vi "Begin.vi"(8 "error in":errorcluster) -> (0 "error out":errorcluster)   [LabVIEW 2020]
doc: "Called before other user functions, this VI can be used to open I/O refnums, load in file data, and do general program initialization. Notice that the <B>error out</B> terminal is simply used for data flow. Wiring it to other structures or subVIs ensures that this VI runs first."
uses:
  <vilib>/Rock Robotics/WPI/DriverStation/WPI_DriverStationRobotMode2.ctl
  <vilib>/Rock Robotics/WPI/Joystick/WPI_JoystickDeviceEnum.ctl
  <vilib>/Rock Robotics/WPI/SafetyOutput/WPI_SafetyOutputConfigMenu.ctl
  <vilib>/Rock Robotics/WPI/ThirdParty/REV Robotics/SPARK MAX/Typedef/Spark MAX Idle Mode.ctl
  <vilib>/Rock Robotics/SystemInterfaces/DIO/FPGA_DIOChannel.ctl
  <vilib>/Rock Robotics/WPI/Solenoid/WPI_SolenoidChannel.ctl
  <vilib>/Rock Robotics/WPI/Solenoid/WPI_SolenoidValue.ctl
  <vilib>/Rock Robotics/SystemInterfaces/DIO/FPGA_DIOPWMChannel.ctl
  Robot Global Data.vi
  <vilib>/Rock Robotics/Network Tables/NT Write String Array.vi
  <vilib>/Rock Robotics/WPI/Solenoid/WPI_SolenoidOpenDouble.vi
  <vilib>/Rock Robotics/WPI/Utilities/WPI_GetSetVariantRefNum.vi
  <vilib>/Rock Robotics/WPI/Solenoid/WPI_SolenoidSetEnum.vi
  <vilib>/Rock Robotics/WPI/MotorControl/WPI_MotorControlOpen SPARK.vi
  <vilib>/Rock Robotics/WPI/MotorControl/WPI_MotorControlOpen VictorSPX.vi
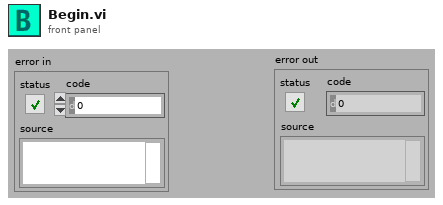
[diagram p1: front panel]
types:
  T1 = typedef "FPGA_DIOPWMChannel.ctl" = enum8{"PWM 0", "PWM 1", "PWM 2", "PWM 3", "PWM 4", "PWM 5", "PWM 6", "PWM 7", "PWM 8", "PWM 9", "PWM MXP 0", "PWM MXP 1", "PWM MXP 2", "PWM MXP 3", "PWM MXP 4", "PWM MXP 5", "PWM MXP 6", "PWM MXP 7", "PWM MXP 8", "PWM MXP 9", "Invalid"}
  T2 = typedef "WPI_SafetyOutputConfigMenu.ctl" = enum16{"Enable", "Disable"}
  T3 = typedef "WPI_SolenoidValue.ctl" = enum16{"Off", "On", "Forward", "Reverse"}
  T4 = typedef "WPI_SolenoidChannel.ctl" = enum8{"Solenoid 0", "Solenoid 1", "Solenoid 2", "Solenoid 3", "Solenoid 4", "Solenoid 5", "Solenoid 6", "Solenoid 7", "Solenoid 8", "Solenoid 9", "Solenoid 10", "Solenoid 11", "Solenoid 12", "Solenoid 13", "Solenoid 14", "Solenoid 15", "Invalid"}
  T5 = typedef "Spark MAX Idle Mode.ctl" = enum16{"Coast", "Brake"}
  T6 = typedef "FPGA_DIOChannel.ctl" = enum8{"DIO 0", "DIO 1", "DIO 2", "DIO 3", "DIO 4", "DIO 5", "DIO 6", "DIO 7", "DIO 8", "DIO 9", "DIO MXP 0", "DIO MXP 1", "DIO MXP 2", "DIO MXP 3", "DIO MXP 4", "DIO MXP 5", "DIO MXP 6", "DIO MXP 7", "DIO MXP 8", "DIO MXP 9", "DIO MXP 10", "DIO MXP 11", "DIO MXP 12", "DIO MXP 13", "DIO MXP 14", "DIO MXP 15", "SPI Port CS1", "SPI Port CS2", "SPI Port CS3", "SPI Port MISO", "SPI Port MOSI", "Invalid"}
  T7 = typedef "WPI_JoystickDeviceEnum.ctl" = enum16{"USB 0", "USB 1", "USB 2", "USB 3", "USB 4", "USB 5"}
  T8 = typedef "WPI_DriverStationRobotMode2.ctl" = enum16{"Autonomous Disabled", "Autonomous Enabled", "Teleop Disabled", "Teleop Enabled", "Disconnected", "Finish", "Test Disabled", "Test Enabled", "Emergency Stopped"}
  T9 = typedef "WPI_MotorControlDeviceRef.ctl" = cluster{"DeviceStatus":errorcluster, "Type":T10, "PWM":cluster{"PWM Channel":T1, "DeadBand":T11}, "CAN":cluster{"Device Number":u8, "SetOutput VI Ref":variant, "GetOutput VI Ref":variant, "Enable VI Ref":variant, "Disable VI Ref":variant, "Data":variant}, "Invert":bool, "DIO PWM":cluster{"PWM \"Enable\" Channel":T1, "DIOChannel":T6, "PWM Rate":dbl}}
  T10 = typedef "WPI_MotorControlType.ctl" = enum16{"PWM", "CAN", "DIO PWM"}
  T11 = typedef "WPI_PWMDeadband.ctl" = cluster{"Name":string, "maxPositivePwm":i32, "minPositivePwm":i32, "centerPwm":i32, "maxNegativePwm":i32, "minNegativePwm":i32, "angularRange":u16}
  T12 = typedef "WPI_SolenoidDevRef.ctl" = cluster{"DevStatus":errorcluster, "Pneumatics Control Module":u8, "Forward Solenoid Channel":T4, "Reverse Solenoid Channel":T4}
  T13 = typedef "WPI_JoystickDevRef.ctl" = cluster{"Device":T7}
  T14 = typedef "ADIS16470 Device Reference.ctl" = cluster{"DevStatus":errorcluster, "Hardware Config":T15, "Calibration Complete":refnum<notifier>, "Status Reference":refnum<data-value>, "Data Reference":refnum<data-value>, "Sychronous Process VI":T18, "Cmd FIFO":refnum<k33>, "Source":T19, "Data FIFO":refnum<k33>, "Calibration Time (ms)":u32, "Data Reference":refnum<data-value>}
  T15 = typedef "ADIS16470 Hardware Configuration.ctl" = cluster{"SPI Clock Rate (Hz)":dbl, "IMU SPI Mode (3)":T16, "IMU Reset Pin":T6, "IMU SPI Bus":T17, "IMU Data Ready Pin":T6, "Stall Config":cluster{"Pow2BytesPerRead":u8, "StallTicks":u16, "CsToSclkTicks":u8}}
  T16 = typedef "WPI_SPIMode.ctl" = enum16{"Mode 0 (Clk Idle Low,Sample on Leading)", "Mode 1 (Clk Idle Low,Sample on Trailing)", "Mode 2 (Clk Idle High,Sample on Leading)", "Mode 3 (Clk Idle High,Sample on Trailing)"}
  T17 = typedef "spi_bus.ctl" = enum16{"SPI On-Board, CS0", "SPI On-Board, CS1", "SPI On-Board, CS2", "SPI On-Board, CS3", "SPI MXP", "Invalid"}
  T18 = typedef "ADIS16470 Process.ctl" = refnum<vi>
  T19 = typedef "FPGA_CounterEncoderSourceConvertionLVSourceType.ctl" = cluster{"DevStatus":errorcluster, "AnalogTriggerMode?":bool, "DigitalMode":cluster{"DIO Channel":T20}, "AnalogTriggerMode":cluster{"AnalogTriggerIndex":T21, "OutputType":T22}}
  T20 = typedef "FPGA_DIODigitalSourceChannel.ctl" = enum8{"DIO 0", "DIO 1", "DIO 2", "DIO 3", "DIO 4", "DIO 5", "DIO 6", "DIO 7", "DIO 8", "DIO 9", "DIO MXP 0", "DIO MXP 1", "DIO MXP 2", "DIO MXP 3", "DIO MXP 4", "DIO MXP 5", "DIO MXP 6", "DIO MXP 7", "DIO MXP 8", "DIO MXP 9", "DIO MXP 10", "DIO MXP 11", "DIO MXP 12", "DIO MXP 13", "DIO MXP 14", "DIO MXP 15", "SPI Port CS1", "SPI Port CS2", "SPI Port CS3", "SPI Port MISO", "SPI Port MOSI", "Disabled"}
  T21 = typedef "FPGA_AnalogTriggerIndex.ctl" = enum8{"Trig 0", "Trig 1", "Trig 2", "Trig 3", "Trig 4", "Trig 5", "Trig 6", "Trig 7", "Invalid"}
  T22 = typedef "FPGA_AnalogTriggerOutType.ctl" = enum16{"InWindow", "TriggerState", "Rising", "Falling"}
  T23 = typedef "WPI_DigitalInputDevRef.ctl" = cluster{"DevStatus":errorcluster, "DIO Channel":T6}
  T24 = typedef "WPI_CompressorDevRef.ctl" = cluster{"DevStatus":errorcluster, "Pneumatics Control Module":u8}
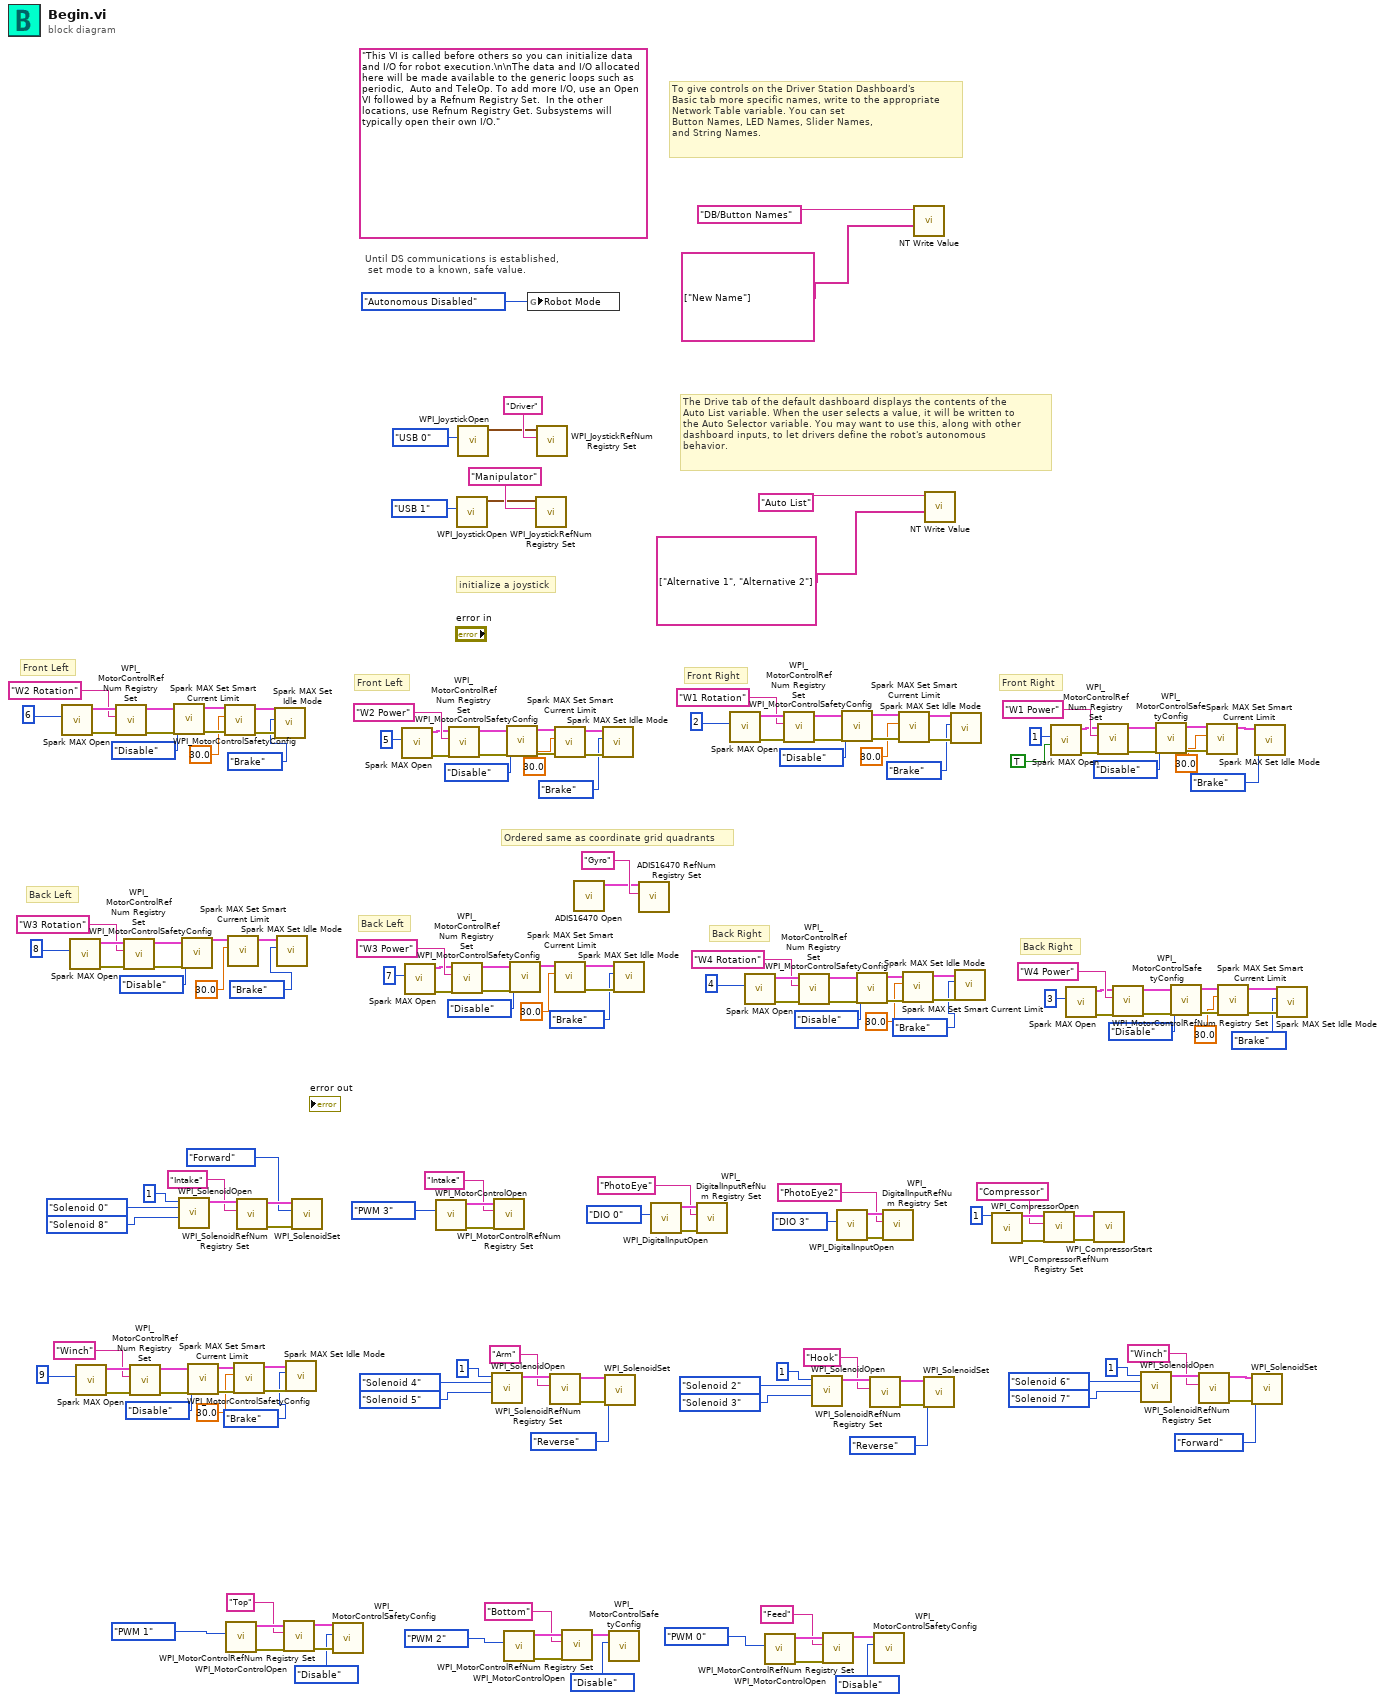
[diagram p0: block diagram]
diagram:
  (unwired) "This VI is called before others so you can initialize data and I/O for robot execution.\n\nThe data and I/O allocated here will be made available to the generic loops such as periodic,  Auto and TeleOp. To add more I/O, use an Open VI followed by a Refnum Registry Set.  In the other locations, use Refnum Registry Get. Subsystems will typically open their own I/O."
  # "Ordered same as coordinate grid quadrants"
  # "Back Right"
  # "Back Right"
  # "Back Left"
  # "Back Left"
  # "Front Left"
  # "Front Left"
  # "Front Right"
  # "Front Right"
  # "The Drive tab of the default dashboard displays the contents of the\nAuto List variable. When the user selects a value, it will be written to\nthe Auto Selector variable. You may want to use this, along with other\ndashboard inputs, to let drivers define the robot's autonomous\nbehavior."
  # "To give controls on the Driver Station Dashboard's\nBasic tab more specific names, write to the appropriate\nNetwork Table variable. You can set\nButton Names, LED Names, Slider Names,\nand String Names."
  # "initialize a joystick"
  # "Until DS communications is established,\n set mode to a known, safe value."
  n1 = call <vilib>:"Spark MAX Open.vi"("Device Number"=u8 6) -> ("error out"=w172:errorcluster, "MotorControlDeviceRef"=w171:T9)  [unwired: 9 in]
  n2 = call <vilib>:"Spark MAX Open.vi"("Device Number"=u8 8) -> ("error out"=w160:errorcluster, "MotorControlDeviceRef"=w159:T9)  [unwired: 9 in]
  n3 = call <vilib>:"Spark MAX Open.vi"("Device Number"=u8 9) -> ("error out"=w68:errorcluster, "MotorControlDeviceRef"=w67:T9)  [unwired: 9 in]
  n4 = call <vilib>:"WPI_MotorControlRefNum Registry Set.vi"("error in (no error)"=w172, "refnum name"="W2 Rotation", "MotorControlDevRef"=w171) -> ("error out"=w170:errorcluster, "MotorControlDevRef"=w108:T9)  [unwired: 7 in]
  n5 = call <vilib>:"WPI_MotorControlRefNum Registry Set.vi"("error in (no error)"=w160, "refnum name"="W3 Rotation", "MotorControlDevRef"=w159) -> ("error out"=w158:errorcluster, "MotorControlDevRef"=w157:T9)  [unwired: 7 in]
  n6 = call <vilib>:"WPI_MotorControlRefNum Registry Set.vi"("error in (no error)"=w68, "refnum name"="Winch", "MotorControlDevRef"=w67) -> ("error out"=w66:errorcluster, "MotorControlDevRef"=w65:T9)  [unwired: 7 in]
  n7 = call <vilib>:"WPI_MotorControlSafetyConfig.vi"("error in (no error)"=w170, "mode"=WPI_SafetyOutputConfigMenu."Disable", "MotorControlDevRef"=w108) -> ("error out"=w111:errorcluster, "MotorControlDevRef"=w110:T9)  [unwired: 7 in]
  n8 = call-poly <vilib>:"WPI_SolenoidOpen.vi"("Reverse Solenoid Channel"=WPI_SolenoidChannel."Solenoid 8", "Forward Solenoid Channel"=WPI_SolenoidChannel."Solenoid 0", "Pneumatics Device (def)"=u8 1) -> ("SolenoidDevRef"=w81:T12)  [unwired: 7 in, 1 out]
  n9 = call <vilib>:"WPI_MotorControlSafetyConfig.vi"("error in (no error)"=w158, "mode"=WPI_SafetyOutputConfigMenu."Disable", "MotorControlDevRef"=w157) -> ("MotorControlDevRef"=w130:T9)  [unwired: 7 in, 1 out]
  n10 = call <vilib>:"WPI_MotorControlSafetyConfig.vi"("error in (no error)"=w66, "mode"=WPI_SafetyOutputConfigMenu."Disable", "MotorControlDevRef"=w65) -> ("error out"=w61:errorcluster, "MotorControlDevRef"=w60:T9)  [unwired: 7 in]
  n11 = call <vilib>:"Spark MAX Set Smart Current Limit.vi"("error in (no error)"=w111, "Primay Current Limit (80A)"=30.0, "MotorControlDeviceRef in"=w110) -> ("error out"=w96:errorcluster, "MotorControlDeviceRef out"=w95:T9)  [unwired: 7 in]
  n12 = call-poly <vilib>:"WPI_MotorControlOpen.vi"("PWM Channel"=FPGA_DIOPWMChannel."PWM 1") -> ("error out"=w20:errorcluster, "MotorControlDeviceRef"=w19:T9)  [unwired: 9 in]
  n13 = call <vilib>:"Spark MAX Set Smart Current Limit.vi"("Primay Current Limit (80A)"=30.0, "MotorControlDeviceRef in"=w130) -> ("MotorControlDeviceRef out"=w97:T9)  [unwired: 8 in, 1 out]
  n14 = call <vilib>:"Spark MAX Set Smart Current Limit.vi"("error in (no error)"=w61, "Primay Current Limit (80A)"=30.0, "MotorControlDeviceRef in"=w60) -> ("error out"=w58:errorcluster, "MotorControlDeviceRef out"=w57:T9)  [unwired: 7 in]
  n15 = call <vilib>:"WPI_SolenoidRefNum Registry Set.vi"("refnum name"="Intake", "SolenoidDevRef"=w81) -> ("error out"=w32:errorcluster, "SolenoidDevRef"=w31:T12)  [unwired: 8 in]
  n16 = call <vilib>:"Spark MAX Set Idle Mode.vi"("error in (no error)"=w96, "Idle Mode"=Spark_MAX_Idle_Mode."Brake", "MotorControlDeviceRef in"=w95) -> ()  [unwired: 7 in, 2 out]
  n17 = call <vilib>:"Spark MAX Set Idle Mode.vi"("Idle Mode"=Spark_MAX_Idle_Mode."Brake", "MotorControlDeviceRef in"=w97) -> ()  [unwired: 8 in, 2 out]
  n18 = call <vilib>:"WPI_MotorControlRefNum Registry Set.vi"("error in (no error)"=w20, "refnum name"="Top", "MotorControlDevRef"=w19) -> ("error out"=w4:errorcluster, "MotorControlDevRef"=w3:T9)  [unwired: 7 in]
  n19 = call <vilib>:"Spark MAX Set Idle Mode.vi"("error in (no error)"=w58, "Idle Mode"=Spark_MAX_Idle_Mode."Brake", "MotorControlDeviceRef in"=w57) -> ()  [unwired: 7 in, 2 out]
  n20 = call-poly <vilib>:"WPI_SolenoidSet.vi"("error in (no error)"=w32, "Value"=WPI_SolenoidValue."Forward", "SolenoidDevRef"=w31) -> ()  [unwired: 7 in, 2 out]
  n21 = call <vilib>:"WPI_MotorControlSafetyConfig.vi"("error in (no error)"=w4, "mode"=WPI_SafetyOutputConfigMenu."Disable", "MotorControlDevRef"=w3) -> ()  [unwired: 7 in, 2 out]
  n22 = call <vilib>:"Spark MAX Open.vi"("Device Number"=u8 5) -> ("error out"=w162:errorcluster, "MotorControlDeviceRef"=w163:T9)  [unwired: 9 in]
  n23 = call <vilib>:"Spark MAX Open.vi"("Device Number"=u8 7) -> ("error out"=w149:errorcluster, "MotorControlDeviceRef"=w150:T9)  [unwired: 9 in]
  n24 = call-poly <vilib>:"WPI_MotorControlOpen.vi"("PWM Channel"=FPGA_DIOPWMChannel."PWM 3") -> ("error out"=w79:errorcluster, "MotorControlDeviceRef"=w78:T9)  [unwired: 9 in]
  n25 = call <vilib>:"WPI_MotorControlRefNum Registry Set.vi"("error in (no error)"=w162, "refnum name"="W2 Power", "MotorControlDevRef"=w163) -> ("error out"=w167:errorcluster, "MotorControlDevRef"=w166:T9)  [unwired: 7 in]
  n26 = call <vilib>:"WPI_MotorControlRefNum Registry Set.vi"("error in (no error)"=w149, "refnum name"="W3 Power", "MotorControlDevRef"=w150) -> ("error out"=w154:errorcluster, "MotorControlDevRef"=w153:T9)  [unwired: 7 in]
  n27 = call <vilib>:"WPI_JoystickOpen.vi"("JoystickDevice"=WPI_JoystickDeviceEnum."USB 1") -> ("JoystickDevRef"=w187:T13)  [unwired: 10 in]
  n28 = call <vilib>:"WPI_JoystickOpen.vi"("JoystickDevice"=WPI_JoystickDeviceEnum."USB 0") -> ("JoystickDevRef"=w194:T13)  [unwired: 10 in]
  n29 = call-poly <vilib>:"WPI_SolenoidOpen.vi"("Reverse Solenoid Channel"=WPI_SolenoidChannel."Solenoid 5", "Forward Solenoid Channel"=WPI_SolenoidChannel."Solenoid 4", "Pneumatics Device (def)"=u8 1) -> ("SolenoidDevRef"=w52:T12)  [unwired: 7 in, 1 out]
  n30 = call <vilib>:"WPI_MotorControlRefNum Registry Set.vi"("error in (no error)"=w79, "refnum name"="Intake", "MotorControlDevRef"=w78) -> ()  [unwired: 7 in, 2 out]
  n31 = call-poly <vilib>:"WPI_MotorControlOpen.vi"("PWM Channel"=FPGA_DIOPWMChannel."PWM 2") -> ("error out"=w16:errorcluster, "MotorControlDeviceRef"=w15:T9)  [unwired: 9 in]
  n32 = call <vilib>:"WPI_MotorControlSafetyConfig.vi"("error in (no error)"=w167, "mode"=WPI_SafetyOutputConfigMenu."Disable", "MotorControlDevRef"=w166) -> ("error out"=w114:errorcluster, "MotorControlDevRef"=w113:T9)  [unwired: 7 in]
  n33 = call <vilib>:"WPI_MotorControlSafetyConfig.vi"("error in (no error)"=w154, "mode"=WPI_SafetyOutputConfigMenu."Disable", "MotorControlDevRef"=w153) -> ("MotorControlDevRef"=w128:T9)  [unwired: 7 in, 1 out]
  n34 = global write "Robot Global Data.vi" "Robot Mode"(WPI_DriverStationRobotMode2."Autonomous Disabled" ("Robot Mode")) -> ()
  n35 = call <vilib>:"WPI_JoystickRefNum Registry Set.vi"("refnum name"="Manipulator", "JoystickDevRef"=w187) -> ()  [unwired: 8 in, 2 out]
  n36 = call <vilib>:"WPI_JoystickRefNum Registry Set.vi"("refnum name"="Driver", "JoystickDevRef"=w194) -> ()  [unwired: 8 in, 2 out]
  n37 = call <vilib>:"WPI_SolenoidRefNum Registry Set.vi"("refnum name"="Arm", "SolenoidDevRef"=w52) -> ("error out"=w29:errorcluster, "SolenoidDevRef"=w28:T12)  [unwired: 8 in]
  n38 = call <vilib>:"Spark MAX Set Smart Current Limit.vi"("error in (no error)"=w114, "Primay Current Limit (80A)"=30.0, "MotorControlDeviceRef in"=w113) -> ("error out"=w100:errorcluster, "MotorControlDeviceRef out"=w99:T9)  [unwired: 7 in]
  n39 = call <vilib>:"Spark MAX Set Smart Current Limit.vi"("Primay Current Limit (80A)"=30.0, "MotorControlDeviceRef in"=w128) -> ("error out"=w102:errorcluster, "MotorControlDeviceRef out"=w101:T9)  [unwired: 8 in]
  n40 = call <vilib>:"WPI_MotorControlRefNum Registry Set.vi"("error in (no error)"=w16, "refnum name"="Bottom", "MotorControlDevRef"=w15) -> ("MotorControlDevRef"=w5:T9)  [unwired: 7 in, 1 out]
  n41 = call <vilib>:"ADIS16470 Open.vi"() -> ("ADIS16470DevRef"=w83:T14)  [unwired: 10 in, 1 out]
  n42 = call <vilib>:"Spark MAX Set Idle Mode.vi"("error in (no error)"=w100, "Idle Mode"=Spark_MAX_Idle_Mode."Brake", "MotorControlDeviceRef in"=w99) -> ()  [unwired: 7 in, 2 out]
  n43 = call-poly <vilib>:"WPI_SolenoidSet.vi"("error in (no error)"=w29, "Value"=WPI_SolenoidValue."Reverse", "SolenoidDevRef"=w28) -> ()  [unwired: 7 in, 2 out]
  n44 = call <vilib>:"WPI_MotorControlSafetyConfig.vi"("mode"=WPI_SafetyOutputConfigMenu."Disable", "MotorControlDevRef"=w5) -> ()  [unwired: 8 in, 2 out]
  n45 = call <vilib>:"Spark MAX Set Idle Mode.vi"("error in (no error)"=w102, "Idle Mode"=Spark_MAX_Idle_Mode."Brake", "MotorControlDeviceRef in"=w101) -> ()  [unwired: 7 in, 2 out]
  n46 = call <vilib>:"ADIS16470 RefNum Registry Set.vi"("refnum name"="Gyro", "ADIS16470DevRef in"=w83) -> ()  [unwired: 8 in, 2 out]
  n47 = call <vilib>:"WPI_DigitalInputOpen.vi"("DIO Channel"=FPGA_DIOChannel."DIO 0") -> ("error out"=w76:errorcluster, "DigitalInputDevRef"=w75:T23)  [unwired: 9 in]
  n48 = call <vilib>:"WPI_DigitalInputRefNum Registry Set.vi"("error in (no error)"=w76, "refnum name"="PhotoEye", "DigitalInputDevRef"=w75) -> ()  [unwired: 7 in, 2 out]
  n49 = call <vilib>:"Spark MAX Open.vi"("Device Number"=u8 2) -> ("error out"=w185:errorcluster, "MotorControlDeviceRef"=w184:T9)  [unwired: 9 in]
  n50 = call <vilib>:"Spark MAX Open.vi"("Device Number"=u8 4) -> ("error out"=w147:errorcluster, "MotorControlDeviceRef"=w146:T9)  [unwired: 9 in]
  n51 = call-poly <vilib>:"WPI_MotorControlOpen.vi"("PWM Channel"=FPGA_DIOPWMChannel."PWM 0") -> ("error out"=w12:errorcluster, "MotorControlDeviceRef"=w11:T9)  [unwired: 9 in]
  n52 = call <vilib>:"WPI_MotorControlRefNum Registry Set.vi"("error in (no error)"=w185, "refnum name"="W1 Rotation", "MotorControlDevRef"=w184) -> ("error out"=w183:errorcluster, "MotorControlDevRef"=w182:T9)  [unwired: 7 in]
  n53 = call <vilib>:"WPI_MotorControlRefNum Registry Set.vi"("error in (no error)"=w147, "refnum name"="W4 Rotation", "MotorControlDevRef"=w146) -> ("error out"=w145:errorcluster, "MotorControlDevRef"=w144:T9)  [unwired: 7 in]
  n54 = call-poly <vilib>:"WPI_SolenoidOpen.vi"("Reverse Solenoid Channel"=WPI_SolenoidChannel."Solenoid 3", "Forward Solenoid Channel"=WPI_SolenoidChannel."Solenoid 2", "Pneumatics Device (def)"=u8 1) -> ("SolenoidDevRef"=w47:T12)  [unwired: 7 in, 1 out]
  n55 = call <vilib>:"WPI_MotorControlRefNum Registry Set.vi"("error in (no error)"=w12, "refnum name"="Feed", "MotorControlDevRef"=w11) -> ("MotorControlDevRef"=w7:T9)  [unwired: 7 in, 1 out]
  n56 = call <vilib>:"WPI_DigitalInputOpen.vi"("DIO Channel"=FPGA_DIOChannel."DIO 3") -> ("error out"=w72:errorcluster, "DigitalInputDevRef"=w71:T23)  [unwired: 9 in]
  n57 = call <vilib>:"WPI_MotorControlSafetyConfig.vi"("error in (no error)"=w183, "mode"=WPI_SafetyOutputConfigMenu."Disable", "MotorControlDevRef"=w182) -> ("error out"=w117:errorcluster, "MotorControlDevRef"=w116:T9)  [unwired: 7 in]
  n58 = call <vilib>:"WPI_MotorControlSafetyConfig.vi"("error in (no error)"=w145, "mode"=WPI_SafetyOutputConfigMenu."Disable", "MotorControlDevRef"=w144) -> ("error out"=w126:errorcluster, "MotorControlDevRef"=w125:T9)  [unwired: 7 in]
  n59 = call <vilib>:"WPI_SolenoidRefNum Registry Set.vi"("refnum name"="Hook", "SolenoidDevRef"=w47) -> ("error out"=w24:errorcluster, "SolenoidDevRef"=w25:T12)  [unwired: 8 in]
  n60 = call <vilib>:"WPI_MotorControlSafetyConfig.vi"("mode"=WPI_SafetyOutputConfigMenu."Disable", "MotorControlDevRef"=w7) -> ()  [unwired: 8 in, 2 out]
  n61 = call <vilib>:"WPI_DigitalInputRefNum Registry Set.vi"("error in (no error)"=w72, "refnum name"="PhotoEye2", "DigitalInputDevRef"=w71) -> ()  [unwired: 7 in, 2 out]
  n62 = call <vilib>:"Spark MAX Set Smart Current Limit.vi"("error in (no error)"=w117, "Primay Current Limit (80A)"=30.0, "MotorControlDeviceRef in"=w116) -> ("error out"=w92:errorcluster, "MotorControlDeviceRef out"=w91:T9)  [unwired: 7 in]
  n63 = call <vilib>:"Spark MAX Set Smart Current Limit.vi"("error in (no error)"=w126, "Primay Current Limit (80A)"=30.0, "MotorControlDeviceRef in"=w125) -> ("error out"=w90:errorcluster, "MotorControlDeviceRef out"=w89:T9)  [unwired: 7 in]
  n64 = call-poly <vilib>:"NT Write Value.vi"("String Array"=string[] ["New Name"], "Name"="DB/Button Names") -> ()  [unwired: 9 in, 1 out]
  n65 = call-poly <vilib>:"WPI_SolenoidSet.vi"("error in (no error)"=w24, "Value"=WPI_SolenoidValue."Reverse", "SolenoidDevRef"=w25) -> ()  [unwired: 7 in, 2 out]
  n66 = call-poly <vilib>:"NT Write Value.vi"("String Array"=string[] ["Alternative 1", "Alternative 2"], "Name"="Auto List") -> ()  [unwired: 9 in, 1 out]
  n67 = call <vilib>:"Spark MAX Set Idle Mode.vi"("error in (no error)"=w92, "Idle Mode"=Spark_MAX_Idle_Mode."Brake", "MotorControlDeviceRef in"=w91) -> ()  [unwired: 7 in, 2 out]
  n68 = call <vilib>:"Spark MAX Set Idle Mode.vi"("error in (no error)"=w90, "Idle Mode"=Spark_MAX_Idle_Mode."Brake", "MotorControlDeviceRef in"=w89) -> ()  [unwired: 7 in, 2 out]
  n69 = call <vilib>:"WPI_CompressorOpen.vi"("Pneumatics device (def)"=u8 1) -> ("CompressorDevRef"=w37:T24, "error out"=w38:errorcluster)  [unwired: 13 in]
  n70 = call <vilib>:"WPI_CompressorRefNum Registry Set.vi"("error in (no error)"=w38, "refnum name"="Compressor", "CompressorDevRef"=w37) -> ("error out"=w36:errorcluster, "CompressorDevRef"=w35:T24)  [unwired: 7 in]
  n71 = call <vilib>:"Spark MAX Open.vi"("Invert"=TRUE, "Device Number"=u8 1) -> ("error out"=w174:errorcluster, "MotorControlDeviceRef"=w175:T9)  [unwired: 8 in]
  n72 = call <vilib>:"Spark MAX Open.vi"("Device Number"=u8 3) -> ("error out"=w136:errorcluster, "MotorControlDeviceRef"=w137:T9)  [unwired: 9 in]
  n73 = call <vilib>:"WPI_CompressorStart.vi"("error in (no error)"=w36, "CompressorDevRef"=w35) -> ()  [unwired: 8 in, 2 out]
  n74 = call <vilib>:"WPI_MotorControlRefNum Registry Set.vi"("error in (no error)"=w174, "refnum name"="W1 Power", "MotorControlDevRef"=w175) -> ("error out"=w179:errorcluster, "MotorControlDevRef"=w178:T9)  [unwired: 7 in]
  n75 = call <vilib>:"WPI_MotorControlRefNum Registry Set.vi"("error in (no error)"=w136, "refnum name"="W4 Power", "MotorControlDevRef"=w137) -> ("error out"=w141:errorcluster, "MotorControlDevRef"=w140:T9)  [unwired: 7 in]
  n76 = call-poly <vilib>:"WPI_SolenoidOpen.vi"("Reverse Solenoid Channel"=WPI_SolenoidChannel."Solenoid 7", "Forward Solenoid Channel"=WPI_SolenoidChannel."Solenoid 6", "Pneumatics Device (def)"=u8 1) -> ("SolenoidDevRef"=w42:T12)  [unwired: 7 in, 1 out]
  n77 = call <vilib>:"WPI_MotorControlSafetyConfig.vi"("error in (no error)"=w179, "mode"=WPI_SafetyOutputConfigMenu."Disable", "MotorControlDevRef"=w178) -> ("error out"=w120:errorcluster, "MotorControlDevRef"=w119:T9)  [unwired: 7 in]
  n78 = call <vilib>:"WPI_MotorControlSafetyConfig.vi"("error in (no error)"=w141, "mode"=WPI_SafetyOutputConfigMenu."Disable", "MotorControlDevRef"=w140) -> ("error out"=w123:errorcluster, "MotorControlDevRef"=w122:T9)  [unwired: 7 in]
  n79 = call <vilib>:"WPI_SolenoidRefNum Registry Set.vi"("refnum name"="Winch", "SolenoidDevRef"=w42) -> ("error out"=w21:errorcluster, "SolenoidDevRef"=w22:T12)  [unwired: 8 in]
  n80 = call <vilib>:"Spark MAX Set Smart Current Limit.vi"("error in (no error)"=w120, "Primay Current Limit (80A)"=30.0, "MotorControlDeviceRef in"=w119) -> ("MotorControlDeviceRef out"=w105:T9)  [unwired: 7 in, 1 out]
  n81 = call <vilib>:"Spark MAX Set Smart Current Limit.vi"("error in (no error)"=w123, "Primay Current Limit (80A)"=30.0, "MotorControlDeviceRef in"=w122) -> ("error out"=w104:errorcluster, "MotorControlDeviceRef out"=w103:T9)  [unwired: 7 in]
  n82 = call-poly <vilib>:"WPI_SolenoidSet.vi"("error in (no error)"=w21, "Value"=WPI_SolenoidValue."Forward", "SolenoidDevRef"=w22) -> ()  [unwired: 7 in, 2 out]
  n83 = call <vilib>:"Spark MAX Set Idle Mode.vi"("Idle Mode"=Spark_MAX_Idle_Mode."Brake", "MotorControlDeviceRef in"=w105) -> ()  [unwired: 8 in, 2 out]
  n84 = call <vilib>:"Spark MAX Set Idle Mode.vi"("error in (no error)"=w104, "Idle Mode"=Spark_MAX_Idle_Mode."Brake", "MotorControlDeviceRef in"=w103) -> ()  [unwired: 7 in, 2 out]
